vi "Programa aula_solda.vi"() -> ()   [LabVIEW 2011]
uses:
  <vilib>/Simulation/Scripting/Companion Diagram/SimConfigNode/SimParams.ctl
  <vilib>/Simulation/Scripting/Companion Diagram/SimConfigNode/_simSolvers.ctl
  <vilib>/Simulation/Implementation/Shared/SIMSCR Execution Mode.ctl
  <vilib>/Platform/TimedLoop/XDataNode/timing_clust.ctl
  <vilib>/Platform/TimedLoop/XDataNode/nitl_modes.ctl
  <vilib>/Platform/TimedLoop/XDataNode/wakeup.ctl
  <vilib>/Simulation/Param Hierarchy/Typedefs/SIMPH Param Control Actions.ctl
  <vilib>/Simulation/Implementation/Shared/NILVSim_FinishedLate.vi
  <vilib>/Simulation/DataSources/Implementation/NILVSim Pulse Generator.llb/SIM Pulse Generator (scalar).vi
  <vilib>/Simulation/Utility/Implementation/SIM Halt.vi
  <vilib>/Simulation/Implementation/Shared/NILVSim_Manager.vi
  <vilib>/Simulation/Implementation/Shared/NILVSim_ParamChanged.vi
  <vilib>/Simulation/Implementation/Shared/NILVSim_FinalizeModel.vi
  <vilib>/Simulation/Implementation/Shared/SIM Unbundle Sim Info.vi
  <vilib>/Simulation/Implementation/Shared/NILVSim_GetModelError.vi
  <vilib>/Simulation/Implementation/Shared/SIM Bundle Sim Info.vi
  <vilib>/Simulation/Implementation/Shared/NILVSim_Initialize.vi
  <vilib>/Simulation/Scripting/Companion Diagram/SimConfigNode/SimDog.xnode
  <vilib>/Platform/TimedLoop/XDataNode/XDataNode.xnode
  <vilib>/Simulation/Implementation/XNodeFramework/SimXNode/SimX.xnode
  <vilib>/Platform/TimedLoop/XDataNode/XDNodeRunTimeDep.lvlib
  <vilib>/Simulation/Implementation/Shared/NI_SIM_Implementation.lvlib
panel:
  out "Pulso":dbl
  out "stop":bool
  in  "Numeric":i32
  in  "Duty Cycle (%)":dbl
  out "Seleção manual de Duty Cycle (%)":bool
  out "Leitura de arquivo":bool
  in  "?":bool
  in  "Período de amostragem (ms)":dbl
  out "Duty Cycle (%)":dbl(knob) scale=0.0..100.0
  in  "Arquivo para Leitura":path
  out "Leitura Arquivo":dbl
  in  "Parar":bool
  out "%  Duty Cycle (AO1) 0)":dbl(graph)
  out "Sinal de Temperatura (°C)":dynamicdata(graph) caption="Sinal de Nível (AI 0)"
  in  "Salvar Dados":path=path "test.lvm" caption="Filename"
  # "Selecione o modo de operação:"
  # "Modo Seleção Manual de Duty Cycle"
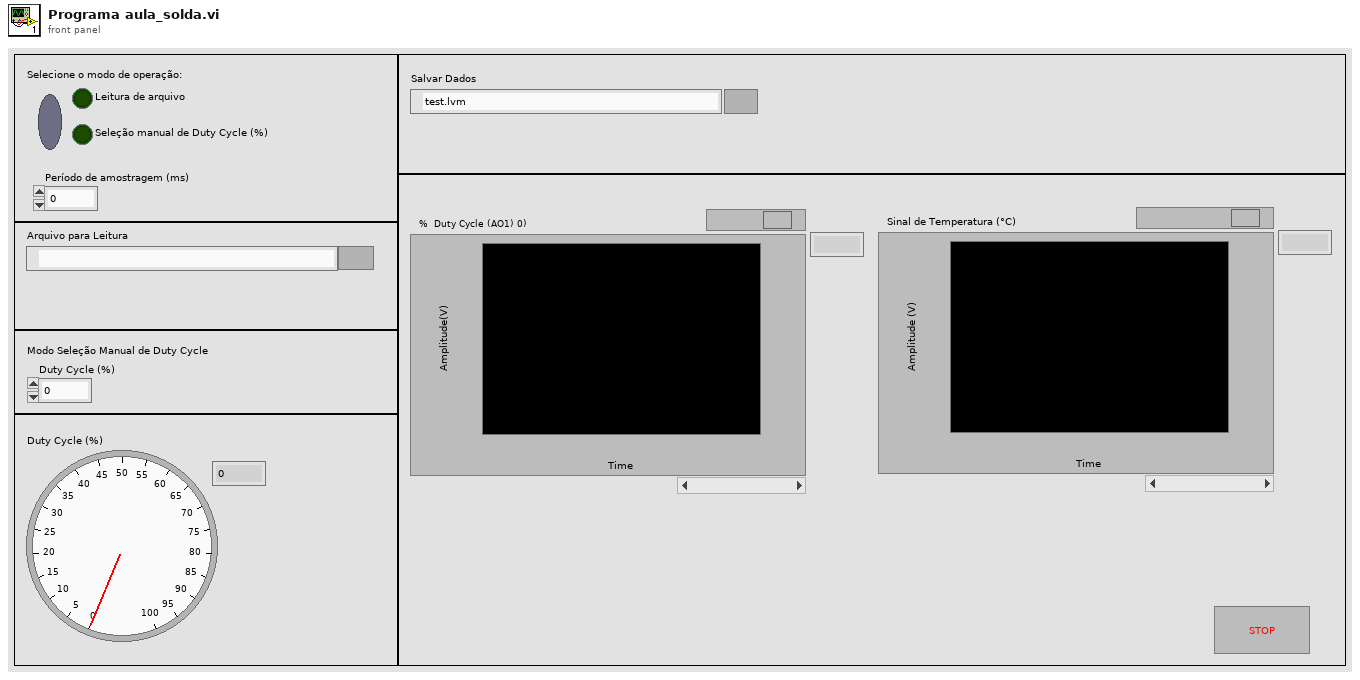
[diagram p1: front panel]
types:
  T1 = enum16{"open", "replace", "create", "open or create", "replace or create", "replace or create with confirmation"}
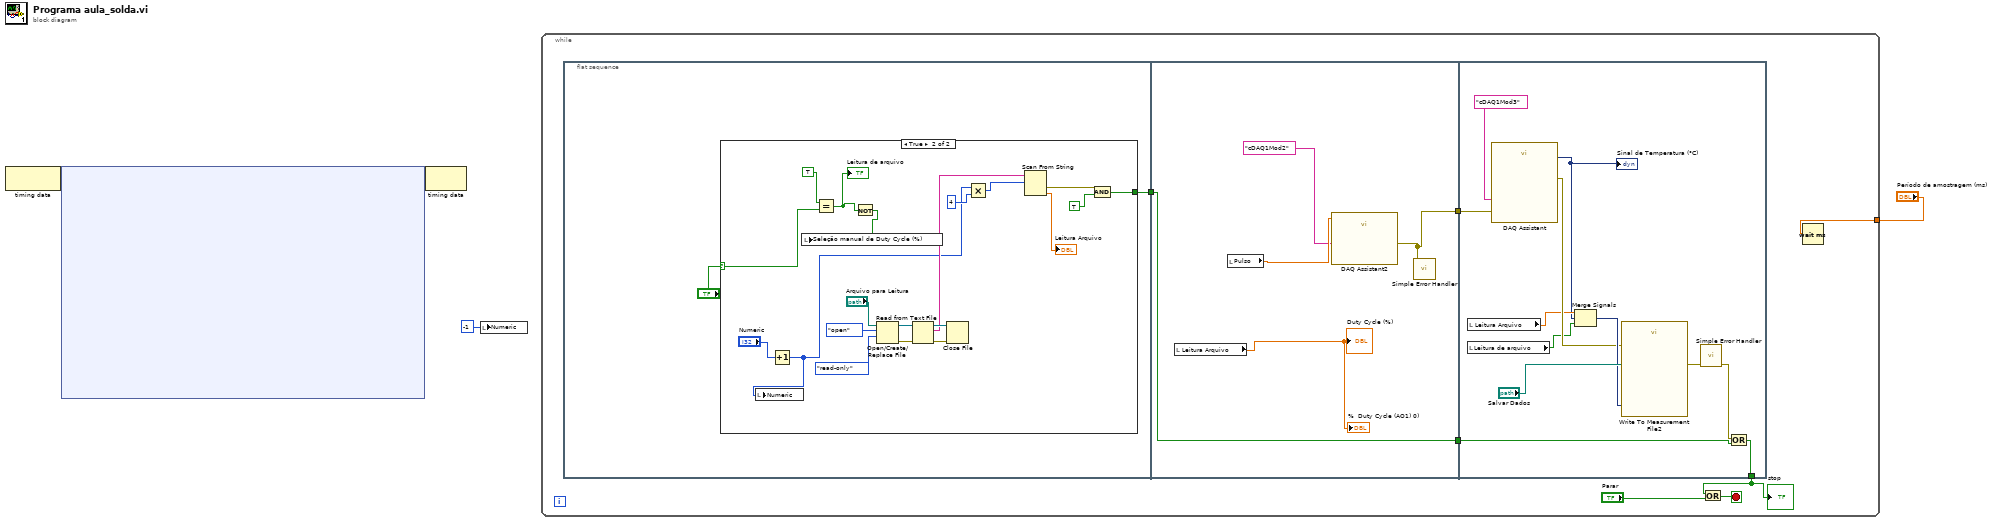
[diagram p0: block diagram]
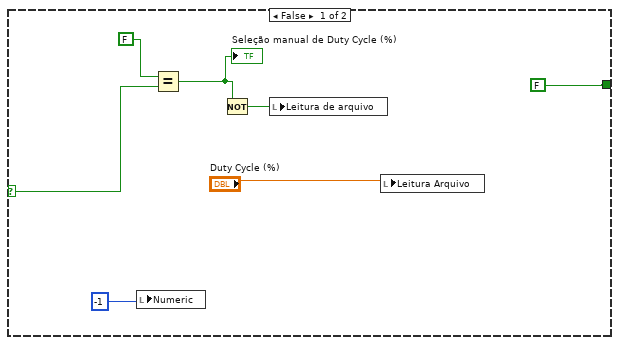
[diagram p2: hidden frame]
diagram:
  n1 = node-c288() -> (w2:variant)  [unwired: 1 in]
  n2 = node-c254 ("Control & Simulation Loop")(w2) -> (w1:variant)
  n3 = node-c288(w1) -> ()  [unwired: 1 out]
  n4 = local write "Numeric"(-1) -> ()
  n5 = while {
    tunnel: "Período de amostragem (ms)" -> [w7]
    stop <- w10 stop-if-true
    n6 = flat-sequence {
      tunnel: [w13] -> w8
      tunnel: [w45] -> w9
      tunnel: w8 -> [w45]
      tunnel: [w41] -> w5
      tunnel: w9 -> [w53]
      tunnel: [w51] -> w6
      tunnel: w5 -> [w46]
      frame #0 {
        n7 = case shown="True" "?" {
          selector: "?" -> [w19 w25]
          tunnel: [FALSE w29] -> w13
          frame False {
            n8 = local write "Numeric"(-1) -> ()
            n9 = Equal?(x=FALSE, y=w19) -> (x = y?=w16:bool)
            "Seleção manual de Duty Cycle (%)" <- w16
            n10 = Not(x=w16) -> (.not. x?=w15:bool)
            n11 = local write "Leitura de arquivo"(w15) -> ()
            n12 = local write "Leitura Arquivo"("Duty Cycle (%)") -> ()
          }
          frame True {
            n13 = Increment(x="Numeric") -> (x+1=w21:i32)
            n14 = local write "Numeric"(w21) -> ()
            n15 = Equal?(x=TRUE, y=w25) -> (x = y?=w24:bool)
            "Leitura de arquivo" <- w24
            n16 = Not(x=w24) -> (.not. x?=w23:bool)
            n17 = local write "Seleção manual de Duty Cycle (%)"(w23) -> ()
            n18 = Open/Create/Replace File(file path (use dialog)="Arquivo para Leitura", operation (0:open)=T1."open", access (0:read/write)=enum16{"read/write", "read-only", "write-only"}."read-only") -> (refnum out=w34:refnum<file>, error out=w38:errorcluster)  [unwired: 3 in, 1 out]
            n19 = Read from Text File(file (use dialog)=w34, error in=w38) -> (refnum out=w40:refnum<file>, text=w33:string, error out=w39:errorcluster)  [unwired: 2 in, 1 out]
            n20 = Close File(refnum=w40, error in=w39) -> ()  [unwired: 2 out]
            n21 = Multiply(x=w21, y=4) -> (x*y=w32:i32)
            n22 = Scan From String(input string=w33, initial scan location=w32) -> (error out=w28:errorcluster, output 1=→"Leitura Arquivo":dbl)  [unwired: 3 in, 2 out]
            n23 = And(x=w28, y=TRUE) -> (x .and. y?=w29:bool)
          }
        }
      }
      frame #1 {
        n24 = local read "Leitura Arquivo"() -> (→"Duty Cycle (%)" →"%  Duty Cycle (AO1) 0)":dbl)
        n25 = local read "Pulso"() -> (w43:dbl)
        n26 = call "DAQ Assistant2"("data"=w43, "device name"="cDAQ1Mod2") -> ("error out"=w41:errorcluster)  [unwired: 16 in, 1 out]
        n27 = call <vilib>:"Simple Error Handler.vi"("error in (no error)"=w41) -> ()  [unwired: 4 in, 5 out]
      }
      frame #2 {
        n28 = local read "Leitura de arquivo"() -> (w49:bool)
        n29 = local read "Leitura Arquivo"() -> (w50:dbl)
        n30 = call "DAQ Assistant"("error in"=w46, "device name"="cDAQ1Mod3") -> ("data"=w48:dynamicdata, "error out"=w55:errorcluster)  [unwired: 14 in, 2 out]
        "Sinal de Temperatura (°C)" <- w48
        n31 = Merge Signals(w50, w48, w49) -> (w56:dynamicdata)
        n32 = call "Write To Measurement File2"("Signals"=w56, "error in (no error)"=w55, "Filename"="Salvar Dados") -> ("error out"=w54:errorcluster)  [unwired: 14 in, 2 out]
        n33 = call <vilib>:"Simple Error Handler.vi"("error in (no error)"=w54) -> ("error out"=w52:errorcluster)  [unwired: 4 in, 4 out]
        n34 = Or(x=w52, y=w53) -> (x .or. y?=w51:bool)
      }
    }
    n35 = Or(x=w6, y="Parar") -> (x .or. y?=w10:bool)
    n36 = Wait (ms)(milliseconds to wait=w7) -> ()  [unwired: 1 out]
    "stop" <- w6
  }
